vi "DoneMessageBroker.vi"(8 "error in (no error)":errorcluster, 11 "Message Broker Interface Ref in":refnum<class "Message Broker Interface Ref.lvclass">) -> (0 "error out":errorcluster, 3 "Message Broker Interface Ref out":refnum<class "Message Broker Interface Ref.lvclass">)   [LabVIEW 2016, in "Stream Mediator.lvlib" / "Message Broker Interface Ref.lvclass"]
doc: "--\nCopyright © 2017 Composed SystemsI All rights reserved.\n\nAuthor: Jon McBee <jon.mcbee@composed.io>\n\nThis library is provided \"AS IS\" ,WITHOUT WARRANTIES OR\nCONDITIONS OF ANY KIND, either express or implied.\n\nComposed Systems -- composed.io\n\nStream 0.0.1.1\nJon McBee - Composed Systems\nCopyright (c) 2017, Composed Systems"
uses:
  <userlib>/Composed Systems/Stream/Mediator/Classes/Message Broker Interface Ref/Message Broker Interface Ref.lvclass
  <userlib>/Composed Systems/Stream/Mediator/Classes/Message Broker Interface Ref/Message Broker Interface Ref.lvclass/Message Broker Interface Ref.ctl
  <userlib>/Composed Systems/Stream/Mediator/Classes/Message Broker/Message Broker.lvclass
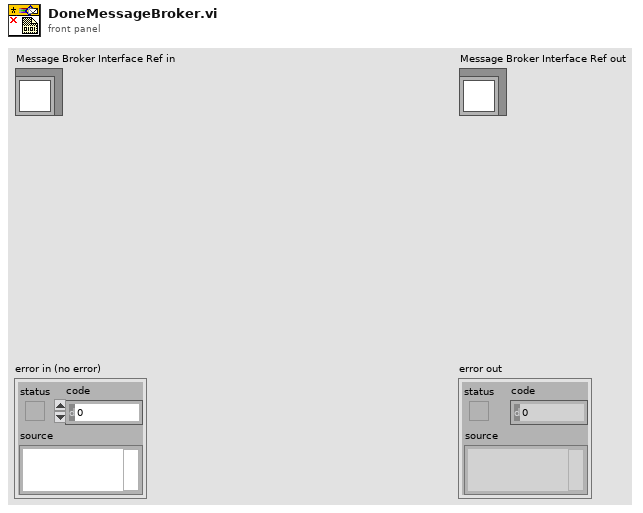
[diagram p1: front panel]
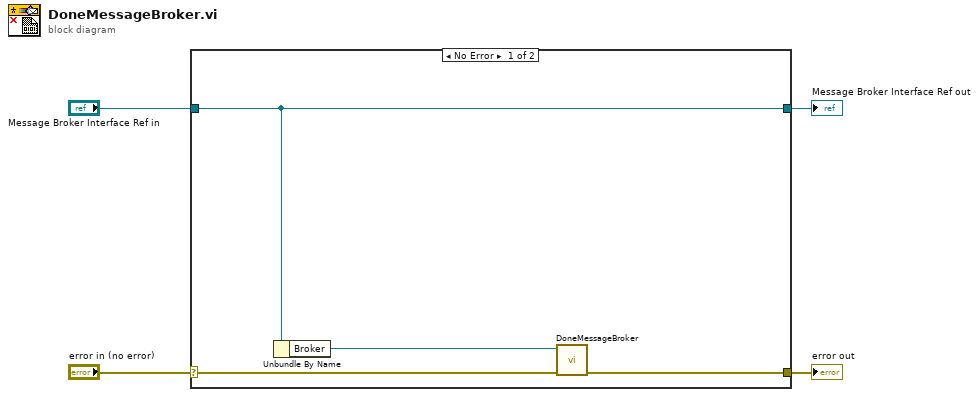
[diagram p0: block diagram]
diagram:
  n1 = case shown="No Error" "error in (no error)" {
    selector: "error in (no error)" -> [w7 w10]
    tunnel: [w6 w10] -> w3
    tunnel: [w8 w9] -> w1
    tunnel: "Message Broker Interface Ref in" -> [w8 w9]
    frame No Error {
      n2 = Unbundle By Name(w8) -> ("Broker"=w5:refnum<data-value>)
      n3 = call <userlib>:"DoneMessageBroker.vi"("error in (no error)"=w7, "Message Broker Ref"=w5) -> ("error out"=w6:errorcluster)  [unwired: 9 in]
    }
    frame Error {
    }
  }
  "error out" <- w3
  "Message Broker Interface Ref out" <- w1
